vi "LV diagram objs.vi"() -> ()   [LabVIEW 2012]
uses:
  <vilib>/_script/All Supported PropertiesOrMethods TypeDefs/ASC_ArrayOfUniqueIDStringParentIDStringName.ctl
  <vilib>/_script/All Supported PropertiesOrMethods TypeDefs/ASC_UniqueIDStringParentIDStringName.ctl
panel:
  out "Array 5":cluster{i32, "AllTypes[]":T1, "Type":T2}[](array[cluster])
  out "Array 4":cluster{i32, refnum<vi>}[](array[cluster])
  out "const":T3(array[cluster])
  out "Array 2":bool[][](array[boolean])
  out "Array":T4(array[cluster])
  out "nodes":T5(array[cluster])
  out "SubVIs":T6(array[cluster])
  out "AllObj":T7(array[cluster])
  out "Decorations[]":refnum<vi>[](array[refnum])
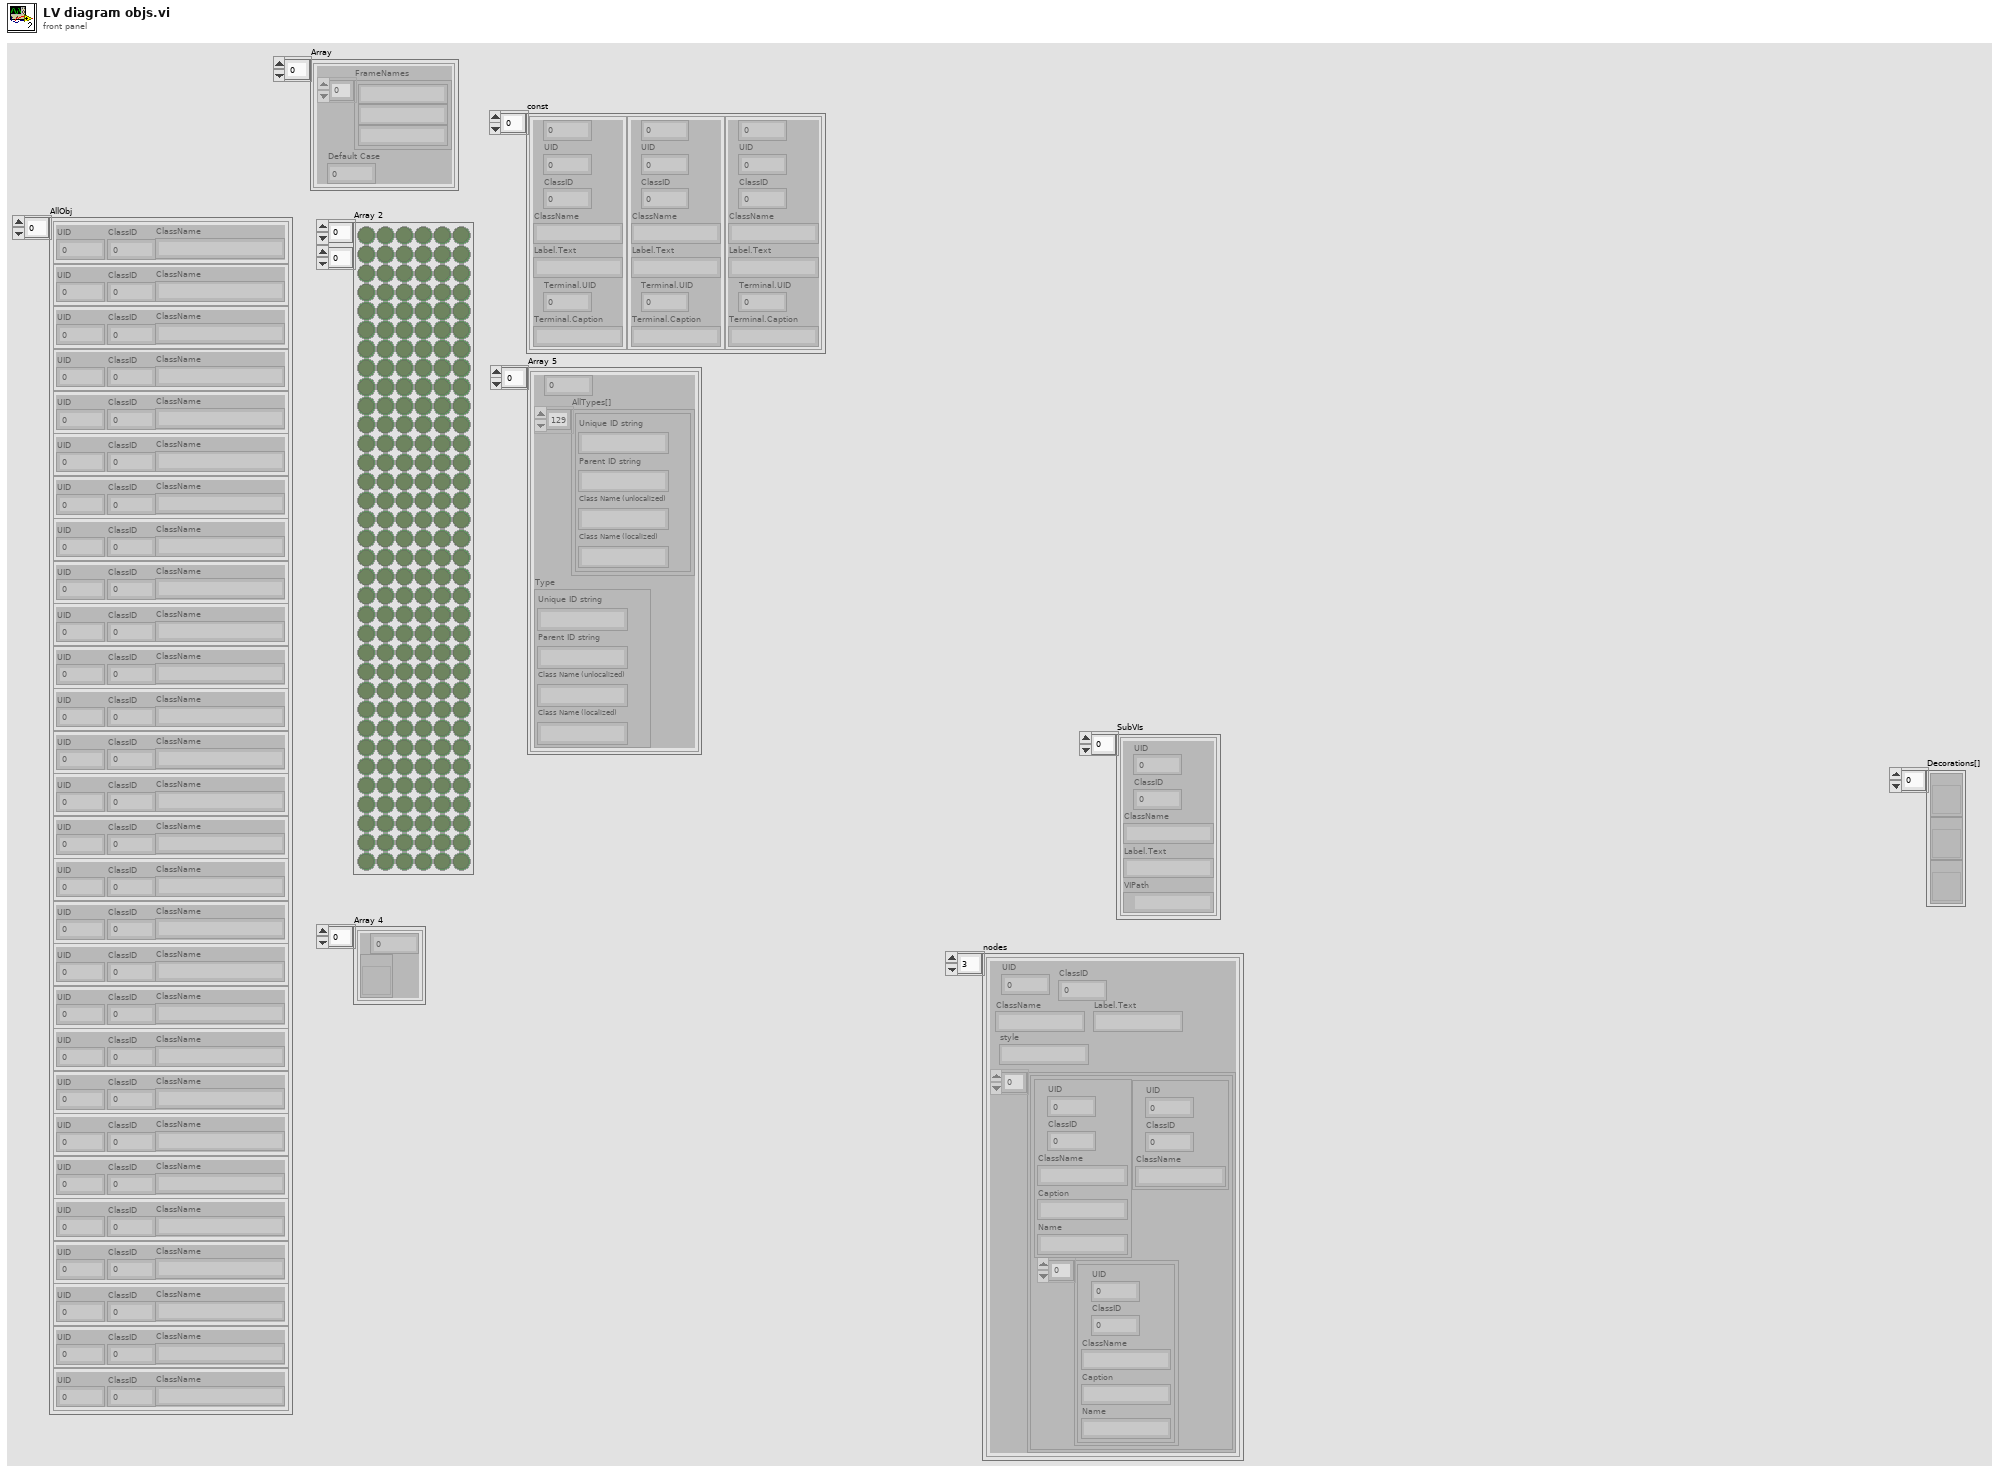
[diagram p1: front panel]
types:
  T1 = typedef "ASC_ArrayOfUniqueIDStringParentIDStringName.ctl" = T2[]
  T2 = typedef "ASC_UniqueIDStringParentIDStringName.ctl" = cluster{"Unique ID string":string, "Parent ID string":string, "Class Name (unlocalized)":string, "Class Name (localized)":string}
  T3 = cluster{i32, "UID":i32, "ClassID":u32, "ClassName":string, "Label.Text":string, "Terminal.UID":i32, "Terminal.Caption":string}[]
  T4 = cluster{"FrameNames":string[], "Default Case":i32}[]
  T5 = cluster{"UID":i32, "ClassID":u32, "ClassName":string, "Label.Text":string, "style":string, cluster{cluster{"UID":i32, "ClassID":u32, "ClassName":string, "Caption":string, "Name":string}, cluster{"UID":i32, "ClassID":u32, "ClassName":string}, cluster{"UID":i32, "ClassID":u32, "ClassName":string, "Caption":string, "Name":string}[]}[]}[]
  T6 = cluster{"UID":i32, "ClassID":u32, "ClassName":string, "Label.Text":string, "VIPath":path}[]
  T7 = cluster{"UID":i32, "ClassID":u32, "ClassName":string}[]
  T8 = cluster{"UID":i32, "ClassID":u32, "ClassName":string}
  T9 = cluster{"UID":i32, "ClassID":u32, "ClassName":string, "Caption":string, "Name":string}
  T10 = cluster{cluster{"UID":i32, "ClassID":u32, "ClassName":string, "Caption":string, "Name":string}, cluster{"UID":i32, "ClassID":u32, "ClassName":string}, cluster{"UID":i32, "ClassID":u32, "ClassName":string, "Caption":string, "Name":string}[]}
  T11 = cluster{"UID":i32, "ClassID":u32, "ClassName":string, "Label.Text":string, "Style":string, cluster{cluster{"UID":i32, "ClassID":u32, "ClassName":string, "Caption":string, "Name":string}, cluster{"UID":i32, "ClassID":u32, "ClassName":string}, cluster{"UID":i32, "ClassID":u32, "ClassName":string, "Caption":string, "Name":string}[]}[]}
  T12 = cluster{"UID":i32, "ClassID":u32, "ClassName":string, "Label.Text":string, "VIPath":path}
  T13 = cluster{i32, "UID":i32, "ClassID":u32, "ClassName":string, "Label.Text":string, "Terminal.UID":i32, "Terminal.Caption":string}
  T14 = cluster{"FrameNames":string[], "Default Case":i32}
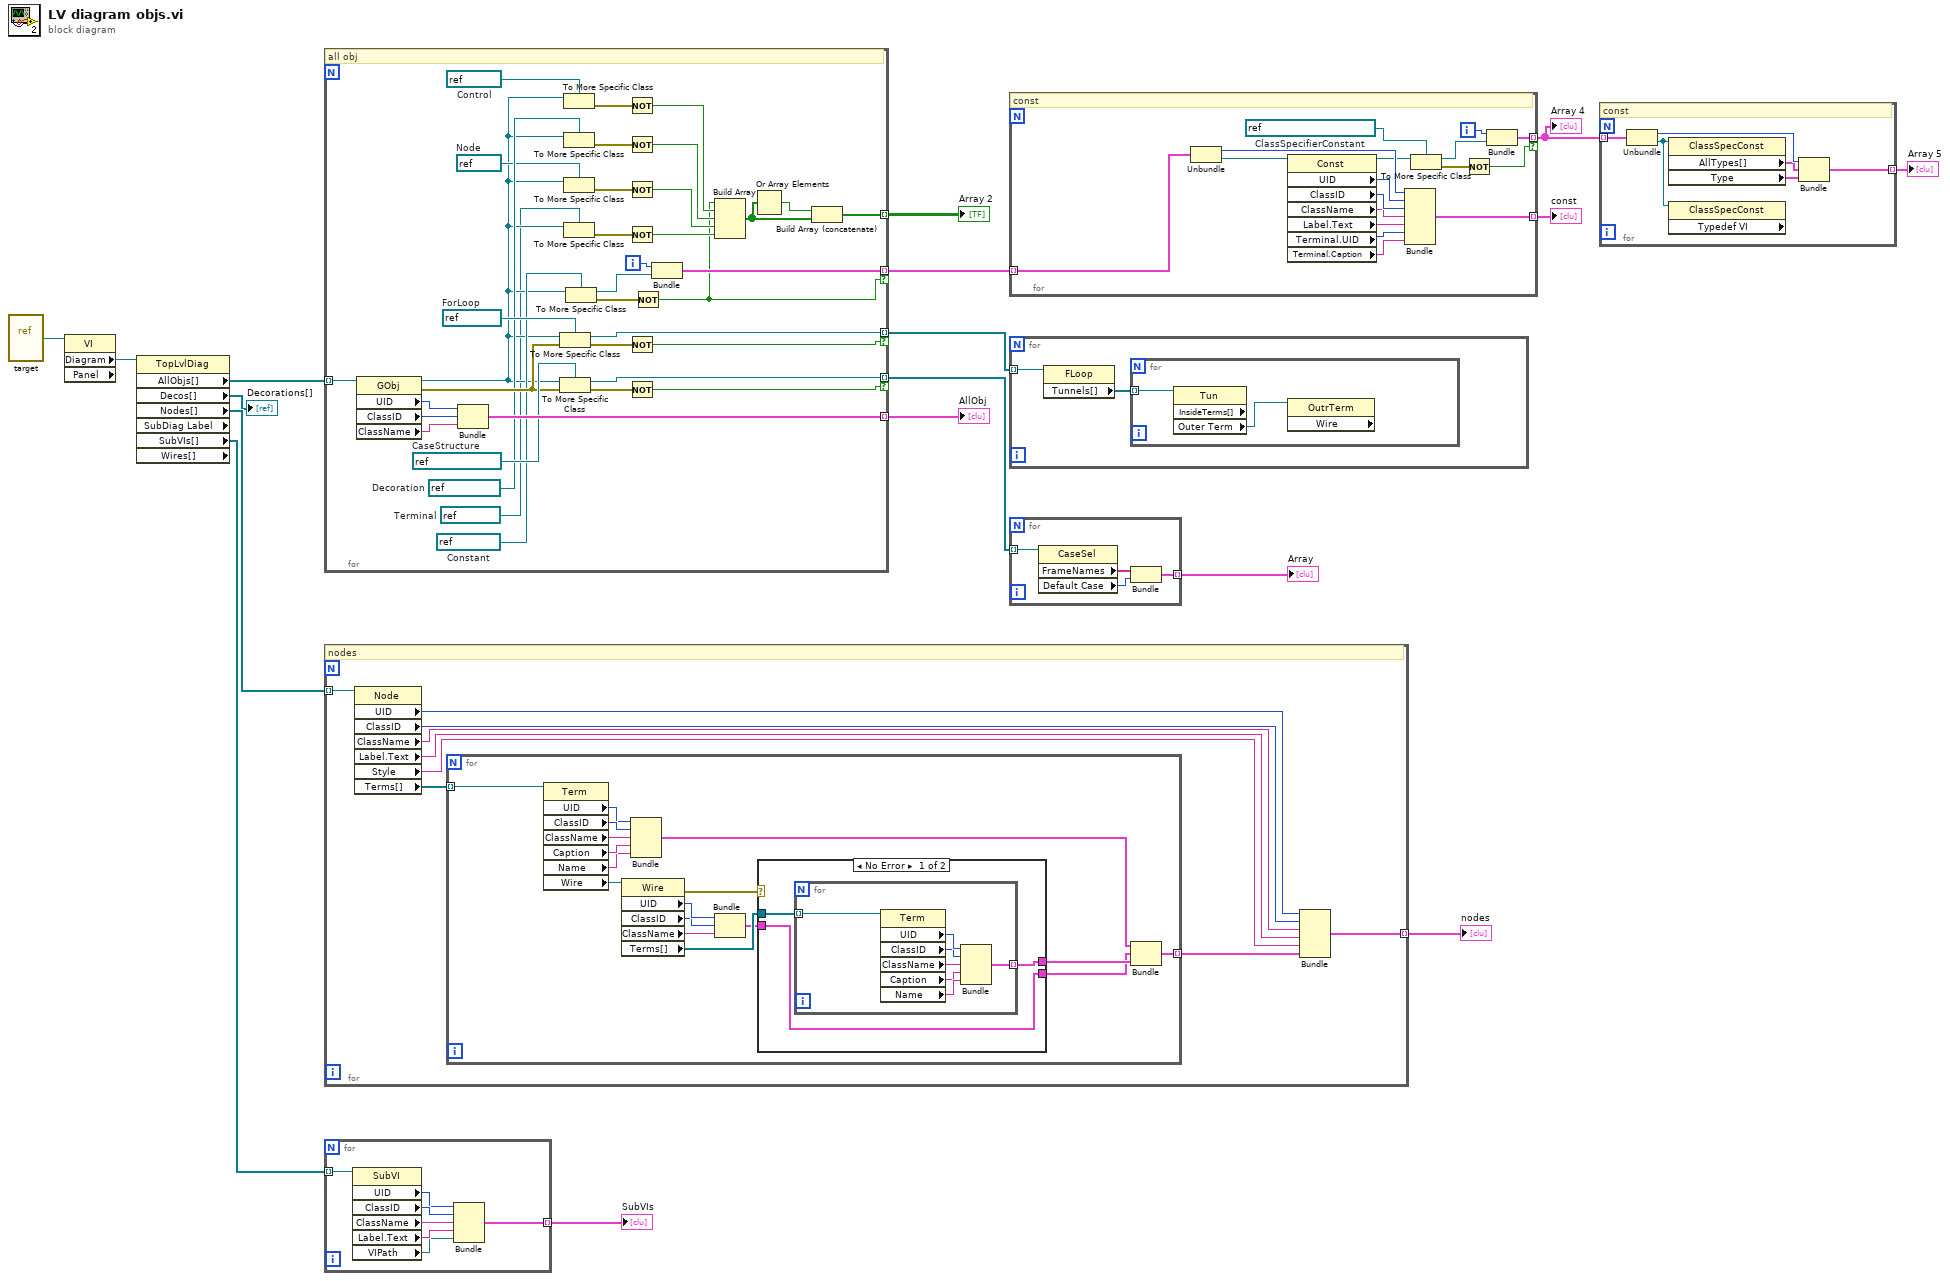
[diagram p0: block diagram]
diagram:
  n1 = vi-ref "target.vi"() -> (w17:refnum<vi>)
  n2 = property class="VI" props=["Diagram", "Panel"](reference=w17) -> ("Diagram"=w16:refnum<vi>)  [unwired: 1 in, 3 out]
  n3 = property class="TopLvlDiag" props=["AllObjs[]", "Decos[]", "Nodes[]", "SubDiag Label", "SubVIs[]", "Wires[]"](reference=w16) -> ("AllObjs[]"=w6:refnum<vi>[], "Decos[]"=→"Decorations[]":refnum<vi>[], "Nodes[]"=w15:refnum<vi>[], "SubVIs[]"=w13:refnum<vi>[])  [unwired: 1 in, 4 out]
  n4 = for {
    tunnel: w6 -> [w42] mode=indexing
    tunnel: [w51] -> w12 mode=indexing
    tunnel: [w48] -> w9 mode=indexing if=w32
    tunnel: [w44] -> w7 mode=indexing if=w33
    tunnel: [w18] -> w5 mode=indexing
    tunnel: [w22] -> w4 mode=indexing if=w21
    i -> [w24]
    w27 = refnum<vi> refnum  # Terminal
    w38 = refnum<vi> refnum  # Node
    w39 = refnum<vi> refnum  # Decoration
    w40 = refnum<vi> refnum  # Control
    w41 = refnum<vi> refnum  # Constant
    w46 = refnum<vi> refnum  # ForLoop
    w49 = refnum<vi> refnum  # CaseStructure
    # "all obj"
    n5 = property class="GObj"(reference=w42) -> (reference out=w28:refnum<vi>, error out=w45:errorcluster, "UID"=w50:i32, "ClassID"=w53:u32, "ClassName"=w52:string)  [unwired: 1 in]
    n6 = Bundle("UID"=w50, "ClassID"=w53, "ClassName"=w52) -> (w51:T8)  [unwired: 1 in]
    n7 = To More Specific Class(target class=w46, reference=w28, error in=w45) -> (specific class reference=w44:refnum<vi>, error out=w43:errorcluster)
    n8 = To More Specific Class(target class=w49, reference=w28, error in=w45) -> (specific class reference=w48:refnum<vi>, error out=w47:errorcluster)
    n9 = To More Specific Class(target class=w40, reference=w28) -> (error out=w36:errorcluster)  [unwired: 1 in, 1 out]
    n10 = To More Specific Class(target class=w39, reference=w28) -> (error out=w35:errorcluster)  [unwired: 1 in, 1 out]
    n11 = To More Specific Class(target class=w38, reference=w28) -> (error out=w34:errorcluster)  [unwired: 1 in, 1 out]
    n12 = To More Specific Class(target class=w27, reference=w28) -> (error out=w26:errorcluster)  [unwired: 1 in, 1 out]
    n13 = To More Specific Class(target class=w41, reference=w28) -> (specific class reference=w23:refnum<vi>, error out=w37:errorcluster)  [unwired: 1 in]
    n14 = Not(x=w36) -> (.not. x?=w31:bool)
    n15 = Not(x=w35) -> (.not. x?=w30:bool)
    n16 = Not(x=w34) -> (.not. x?=w29:bool)
    n17 = Not(x=w26) -> (.not. x?=w25:bool)
    n18 = Not(x=w43) -> (.not. x?=w33:bool)
    n19 = Not(x=w47) -> (.not. x?=w32:bool)
    n20 = Not(x=w37) -> (.not. x?=w21:bool)
    n21 = Bundle(w24, w23) -> (w22:cluster{i32, refnum<vi>})  [unwired: 1 in]
    n22 = Build Array(w21, w31, w30, w29, w25) -> (w20:bool[])
    n23 = Or Array Elements(Boolean array=w20) -> (logical OR=w19:bool)
    n24 = Build Array (concatenate)(w19, w20) -> (w18:bool[])
  }
  "AllObj" <- w12
  "Array 2" <- w5
  n25 = for {
    tunnel: w15 -> [w57] mode=indexing
    tunnel: [w60] -> w10 mode=indexing
    # "nodes"
    n26 = property class="Node"(reference=w57) -> ("UID"=w56:i32, "ClassID"=w62:u32, "ClassName"=w61:string, "Label.Text"=w59:string, "Style"=w54:string, "Terms[]"=w58:refnum<vi>[])  [unwired: 1 in, 2 out]
    n27 = for {
      tunnel: w58 -> [w79] mode=indexing
      tunnel: [w67] -> w55 mode=indexing
      n28 = property class="Term"(reference=w79) -> ("UID"=w74:i32, "ClassID"=w78:u32, "ClassName"=w77:string, "Caption"=w76:string, "Name"=w75:string, "Wire"=w73:refnum<vi>)  [unwired: 1 in, 2 out]
      n29 = property class="Wire"(reference=w73) -> (error out=w63:errorcluster, "UID"=w72:i32, "ClassID"=w71:u32, "ClassName"=w70:string, "Terms[]"=w69:refnum<vi>[])  [unwired: 1 in, 1 out]
      n30 = Bundle("UID"=w74, "ClassID"=w78, "ClassName"=w77, "Caption"=w76, "Name"=w75) -> (w68:T9)  [unwired: 1 in]
      n31 = Bundle("UID"=w72, "ClassID"=w71, "ClassName"=w70) -> (w65:T8)  [unwired: 1 in]
      n32 = case shown="No Error" w63 {
        tunnel: w69 -> [w82 _]
        tunnel: [w81 _] -> w66
        tunnel: w65 -> [w80 _]
        tunnel: [w80 _] -> w64
        frame No Error {
          n33 = for {
            tunnel: w82 -> [w84] mode=indexing
            tunnel: [w83] -> w81 mode=indexing
            n34 = property class="Term"(reference=w84) -> ("UID"=w89:i32, "ClassID"=w85:u32, "ClassName"=w86:string, "Caption"=w87:string, "Name"=w88:string)  [unwired: 1 in, 2 out]
            n35 = Bundle("UID"=w89, "ClassID"=w85, "ClassName"=w86, "Caption"=w87, "Name"=w88) -> (w83:T9)  [unwired: 1 in]
          }
        }
        frame Error {
        }
      }
      n36 = Bundle(w68, w64, w66) -> (w67:T10)  [unwired: 1 in]
    }
    n37 = Bundle("UID"=w56, "ClassID"=w62, "ClassName"=w61, "Label.Text"=w59, "Style"=w54, w55) -> (w60:T11)  [unwired: 1 in]
  }
  "nodes" <- w10
  n38 = for {
    tunnel: w13 -> [w96] mode=indexing
    tunnel: [w93] -> w11 mode=indexing
    n39 = property class="SubVI"(reference=w96) -> ("UID"=w90:i32, "ClassID"=w95:u32, "ClassName"=w94:string, "Label.Text"=w92:string, "VIPath"=w91:path)  [unwired: 1 in, 2 out]
    n40 = Bundle("UID"=w90, "ClassID"=w95, "ClassName"=w94, "Label.Text"=w92, "VIPath"=w91) -> (w93:T12)  [unwired: 1 in]
  }
  "SubVIs" <- w11
  n41 = for {
    tunnel: w4 -> [w113] mode=indexing
    tunnel: [w104] -> w3 mode=indexing
    tunnel: [w99] -> w2 mode=indexing if=w98
    i -> [w100]
    w103 = refnum<vi> refnum  # ClassSpecifierConstant
    # "const"
    n42 = Unbundle(w113) -> (w111:i32, w112:refnum<vi>)
    n43 = property class="Const"(reference=w112) -> (reference out=w102:refnum<vi>, "UID"=w110:i32, "ClassID"=w109:u32, "ClassName"=w108:string, "Label.Text"=w107:string, "Terminal.UID"=w106:i32, "Terminal.Caption"=w105:string)  [unwired: 1 in, 1 out]
    n44 = Bundle(w111, "UID"=w110, "ClassID"=w109, "ClassName"=w108, "Label.Text"=w107, "Terminal.UID"=w106, "Terminal.Caption"=w105) -> (w104:T13)  [unwired: 1 in]
    n45 = To More Specific Class(target class=w103, reference=w102) -> (specific class reference=w97:refnum<vi>, error out=w101:errorcluster)  [unwired: 1 in]
    n46 = Not(x=w101) -> (.not. x?=w98:bool)
    n47 = Bundle(w100, w97) -> (w99:cluster{i32, refnum<vi>})  [unwired: 1 in]
  }
  "const" <- w3
  "Array 4" <- w2
  n48 = for {
    tunnel: w7 -> [w115] mode=indexing
    n49 = property class="FLoop"(reference=w115) -> ("Tunnels[]"=w114:refnum<vi>[])  [unwired: 1 in, 2 out]
    n50 = for {
      tunnel: w114 -> [w117] mode=indexing
      n51 = property class="Tun" props=["InsideTerms[]", "Outer Term"](reference=w117) -> ("Outer Term"=w116:refnum<vi>)  [unwired: 1 in, 3 out]
      n52 = property class="OutrTerm" props=["Wire"](reference=w116) -> ()  [unwired: 1 in, 3 out]
    }
  }
  n53 = for {
    tunnel: w9 -> [w121] mode=indexing
    tunnel: [w118] -> w8 mode=indexing
    n54 = property class="CaseSel"(reference=w121) -> ("FrameNames"=w120:string[], "Default Case"=w119:i32)  [unwired: 1 in, 2 out]
    n55 = Bundle("FrameNames"=w120, "Default Case"=w119) -> (w118:T14)  [unwired: 1 in]
  }
  "Array" <- w8
  n56 = for {
    tunnel: w2 -> [w127] mode=indexing
    tunnel: [w123] -> w1 mode=indexing
    # "const"
    n57 = Unbundle(w127) -> (w126:i32, w122:refnum<vi>)
    n58 = property class="ClassSpecConst"(reference=w122) -> ("AllTypes[]"=w125:T1, "Type"=w124:T2)  [unwired: 1 in, 2 out]
    n59 = property class="ClassSpecConst" props=["Typedef VI"](reference=w122) -> ()  [unwired: 1 in, 3 out]
    n60 = Bundle(w126, "AllTypes[]"=w125, "Type"=w124) -> (w123:cluster{i32, "AllTypes[]":T1, "Type":T2})  [unwired: 1 in]
  }
  "Array 5" <- w1
